vi "_Set All DAC Values.vi"(4 "Record Values (F)":bool, 5 "Load DAC(T)":bool=TRUE, 6 "DAC Value Offset (70)":u16=70, 7 "Channel ID Offset (10)":u16=10, 8 "# of Active Channels":u16) -> ()   [LabVIEW 2015]
uses:
  <vilib>/rvi/Memory/Memory_Emulation/nirvimemoryEmulation.vi
  <vilib>/rvi/Memory/Memory_Emulation/nirvimemoryFastEmulation.vi
  <vilib>/rvi/DataTransferAndStorage/Container/Common/niFpgaContainerGetUniqueNameForEmu.vi
  <vilib>/rvi/Memory/Memory_Emulation/niFpgaMemoryEmulationCacheClearOnFirstRun.vi
  <vilib>/rvi/Memory/Memory_Emulation/nirvimemoryEmulationManagerCache_MakeExclusive.vi
  <vilib>/rvi/Memory/Memory_Emulation/niFpgaMemoryEmulationValidateCache.vi
  <vilib>/rvi/Memory/Memory_Emulation/nirvimemoryEmulationManagerCache_InsertValue.vi
  <vilib>/Utility/error.llb/Clear Errors.vi
  <vilib>/rvi/Memory/Memory_Emulation/nirvimemoryEmulationManagerCache_ReleaseExclusive.vi
  <vilib>/rvi/Memory/Memory_Emulation/nirvimemoryEmulationManagerCache_GetValue.vi
  <vilib>/rvi/Emulation/niFpgaEmulationIsFPGAContextNoSignature.vi
  <vilib>/rvi/Emulation/niFpgaSctlEmulationGetInTimedLoop.vi
  <vilib>/rvi/Memory/Memory_Emulation/nirvimemoryEmulationManagerCache_SetValue.vi
  <vilib>/rvi/Emulation/niFpgaSctlEmulationResourceMgr.vi
  <vilib>/rvi/DataTransferAndStorage/Container/XNode/niFpgaContainer.xnode
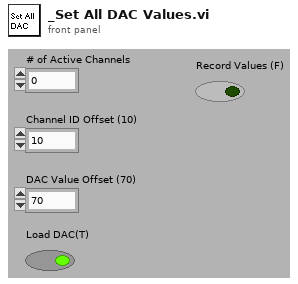
[diagram p1: front panel]
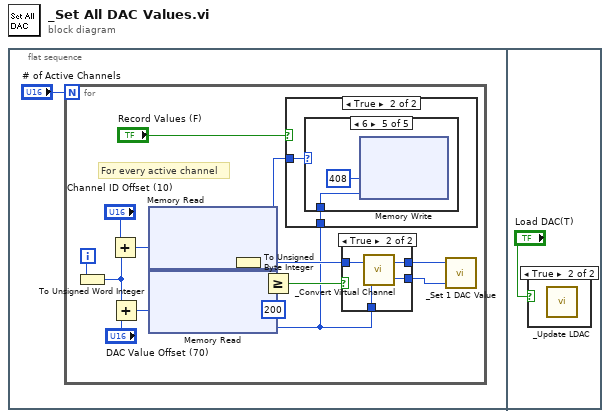
[diagram p0: block diagram]
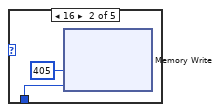
[diagram p4: hidden frame]
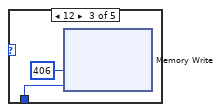
[diagram p5: hidden frame]
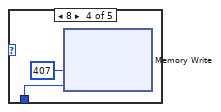
[diagram p6: hidden frame]
diagram:
  n1 = flat-sequence {
    frame #0 {
      n2 = for {
        N: "# of Active Channels" -> [_]
        i -> [w15]
        # "For every active channel"
        n3 = To Unsigned Word Integer(number=w15) -> (unsigned 16bit integer=w11:u16)
        n4 = Add(x="Channel ID Offset (10)", y=w11) -> (x+y=w9:u16)
        n5 = Add(x=w11, y="DAC Value Offset (70)") -> (x+y=w12:u16)
        n6 = xnode ("Memory Read")("Address"=w9) -> ("Data"=w10:u32)  [unwired: 1 in, 1 out]
        n7 = xnode ("Memory Read")("Address"=w12) -> ("Data"=w2:u32)  [unwired: 1 in, 1 out]
        n8 = To Unsigned Byte Integer(number=w10) -> (unsigned 8bit integer=w3:u8)
        n9 = Greater Or Equal?(x=w3, y=u8 200) -> (x >= y?=w5:bool)
        n10 = case shown="True" "Record Values (F)" {
          tunnel: w3 -> [_ w17]
          tunnel: w2 -> [_ w16]
          frame False {
          }
          frame True {
            n11 = case shown="6" w17 {
              tunnel: w16 -> [_ w18 w20 w22 w24]
              frame 0, Default {
              }
              frame 16 {
                n12 = xnode ("Memory Write")("Address"=u32 405, "Data"=w18) -> ()  [unwired: 1 in, 1 out]
              }
              frame 12 {
                n13 = xnode ("Memory Write")("Address"=u32 406, "Data"=w20) -> ()  [unwired: 1 in, 1 out]
              }
              frame 8 {
                n14 = xnode ("Memory Write")("Address"=u32 407, "Data"=w22) -> ()  [unwired: 1 in, 1 out]
              }
              frame 6 {
                n15 = xnode ("Memory Write")("Address"=u32 408, "Data"=w24) -> ()  [unwired: 1 in, 1 out]
              }
            }
          }
        }
        n16 = case shown="True" w5 {
          tunnel: [w27 w31] -> w8
          tunnel: w2 -> [w26 w30]
          tunnel: [w26 w29] -> w7
          tunnel: w3 -> [w27 w28]
          frame False {
          }
          frame True {
            n17 = call "_Convert Virtual Channel.vi"("DAC"=w30, "Ch#"=w28) -> ("DAC Out"=w29:u32, "Ch# Out"=w31:u8)
          }
        }
        n18 = call "_Set 1 DAC Value.vi"("DAC"=w7, "Ch#"=w8) -> ()  [unwired: 2 out]
      }
    }
    frame #1 {
      n19 = case shown="True" "Load DAC(T)" {
        frame False {
        }
        frame True {
          n20 = call "_Update LDAC.vi"() -> ()  [unwired: 6 out]
        }
      }
    }
  }
